vi "Green Board Vref.vi"(8 "error in (no error)":errorcluster) -> (0 "Error Out":errorcluster[](array[cluster]), 3 "Voltage Readings\n\n        3.3V              15V           2.5V            -15V         5V               24V           1.5v":dbl[](array[numeric]))   [LabVIEW 2022 SP3]
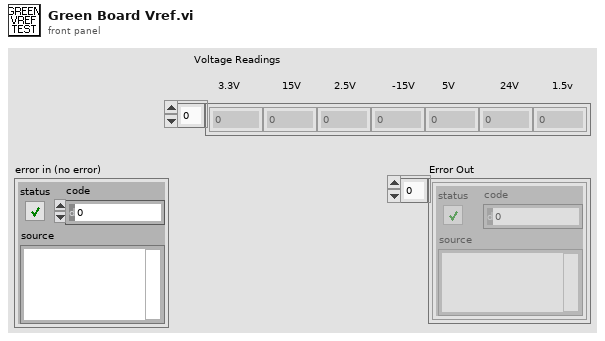
[diagram p1: front panel]
types:
  T1 = cluster{"Enum":enum16{"INVA_ISENSE_U", "INVA_ISENSE_V", "INVA_ISENSE_W", "INVA_UDC", "INVA_TEMP", "HB_ISENSE", "AUX_ISENSE_U", "AUX_ISENSE_V", "AUX_ISENSE_W", "VLINE_AB", "VLINE_BC", "VLINE_CA", "REF_1P5V", "VSENSE_POS_24V", "VSENSE_POS_5V", "VSENSE_NEG_15V", "TEST_POINT", "INVB_ISENSE_U", "INVB_ISENSE_V", "INVB_ISENSE_W", "INVB_UDC", "INVB_TEMP", "HB_TEMP", "AUXA_TEMP", "AUXB_TEMP", "AUXC_TEMP", "VOUT_AB", "VOUT_BC", "VOUT_CA", "REF_2P5V", "VSENSE_POS_15V", "VSENSE_POS_3P3V", "NET_ANALYZER"}}[]
  T2 = enum16{"INVA_ISENSE_U", "INVA_ISENSE_V", "INVA_ISENSE_W", "INVA_UDC", "INVA_TEMP", "HB_ISENSE", "AUX_ISENSE_U", "AUX_ISENSE_V", "AUX_ISENSE_W", "VLINE_AB", "VLINE_BC", "VLINE_CA", "REF_1P5V", "VSENSE_POS_24V", "VSENSE_POS_5V", "VSENSE_NEG_15V", "TEST_POINT", "INVB_ISENSE_U", "INVB_ISENSE_V", "INVB_ISENSE_W", "INVB_UDC", "INVB_TEMP", "HB_TEMP", "AUXA_TEMP", "AUXB_TEMP", "AUXC_TEMP", "VOUT_AB", "VOUT_BC", "VOUT_CA", "REF_2P5V", "VSENSE_POS_15V", "VSENSE_POS_3P3V", "NET_ANALYZER"}
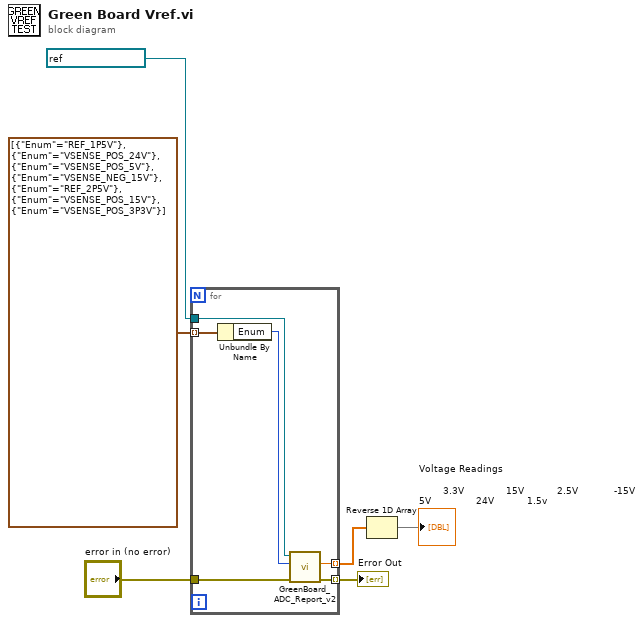
[diagram p0: block diagram]
diagram:
  n1 = for {
    tunnel: T1 [{"Enum"=enum."REF_1P5V"}, {"Enum"=enum."VSENSE_POS_24V"}, {"Enum"=enum."VSENSE_POS_5V"}, {"Enum"=enum."VSENSE_NEG_15V"}, {"Enum"=enum."REF_2P5V"}, {"Enum"=enum."VSENSE_POS_15V"}, {"Enum"=enum."VSENSE_POS_3P3V"}] -> [w12] mode=indexing
    tunnel: [w11] -> w5 mode=indexing
    tunnel: [w10] -> w3 mode=indexing
    tunnel: "error in (no error)" -> [w8]
    tunnel: refnum<visa-resource-name> "ControlBoard" ("ControlBoard VISA") -> [w7]
    n2 = Unbundle By Name(w12) -> ("Enum"=w9:T2)
    n3 = call "GreenBoard_ADC_Report_v2.vi"("error in (no error)"=w8, "Green Board Enum"=w9, "ControlBoard VISA"=w7) -> ("error out"=w10:errorcluster, "Result"=w11:dbl)  [unwired: 5 in, 2 out]
  }
  "Error Out" <- w3
  n4 = Reverse 1D Array(array=w5) -> (reversed array=→"Voltage Readings\n\n        3.3V              15V           2.5V            -15V         5V               24V           1.5v":dbl[])
